vi "Receive Response.vi"(8 "error in":errorcluster, 10 "Response":string, 11 "PS in":refnum<class "Power Supply.lvclass">) -> (0 "error out":errorcluster, 3 "PS out":refnum<class "Power Supply.lvclass">)   [LabVIEW 2019, in "Power Supply.lvlib" / "Power Supply.lvclass"]
uses:
  Power Supply.lvclass
  C:/Program Files (x86)/National Instruments/LabVIEW 2019/vi.lib/ActorFramework/Actor/Actor.lvclass
  Power Supply.lvclass/Power Supply.ctl
  Serial/Serial Messages/Write Msg/Write Msg.lvclass/Write Msg.ctl
  <vilib>/ActorFramework/Message Enqueuer/Message Enqueuer.lvclass/Message Enqueuer.ctl
  <vilib>/ActorFramework/Actor/Actor.lvclass/Actor.ctl
  Power Supply Messages/PS Dataset Msg/PS Dataset Msg.lvclass/PS Dataset Msg.ctl
  <vilib>/ActorFramework/Message Enqueuer/Enqueue.vi
  Serial/Serial Messages/Write Msg/Write Msg.lvclass
  C:/Program Files (x86)/National Instruments/LabVIEW 2019/vi.lib/ActorFramework/Message/Message.lvclass
  Power Supply Messages/PS Dataset Msg/PS Dataset Msg.lvclass
  <userlib>/_MGI/Application Control/MGI Get Value/MGI Get Value (String).vi
  <vilib>/ActorFramework/Message Priority Queue/Priority Enqueue.vi
  <vilib>/ActorFramework/Actor/Actor.lvclass
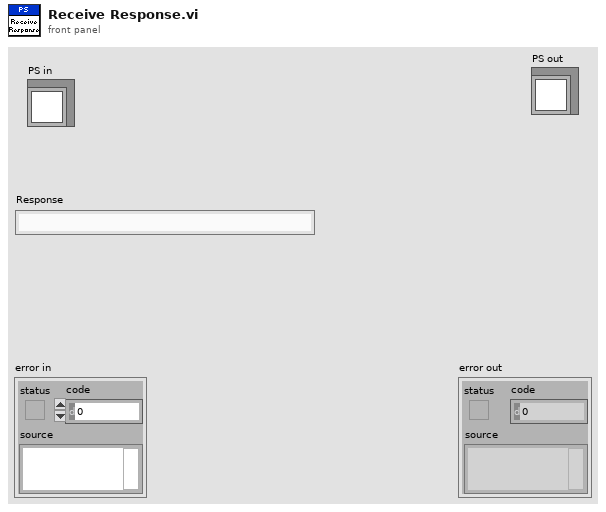
[diagram p1: front panel]
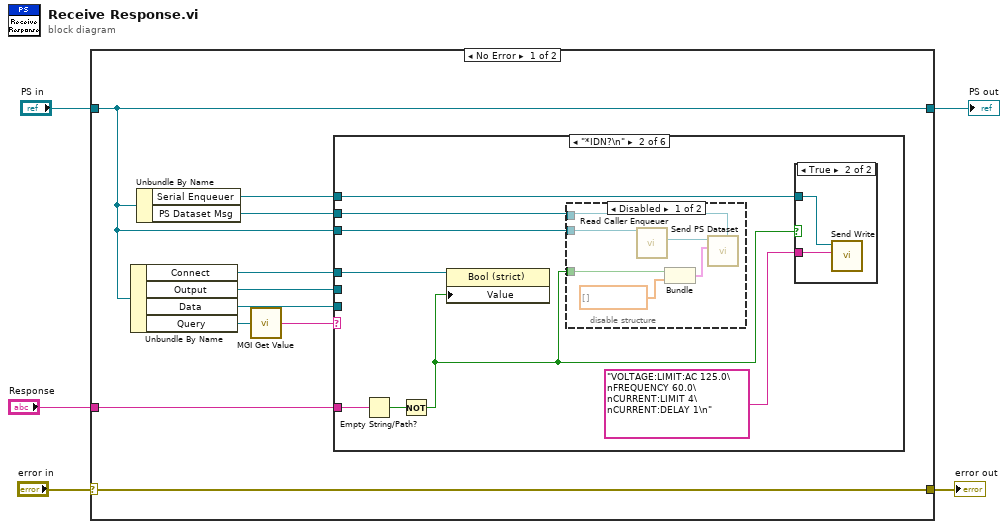
[diagram p0: block diagram]
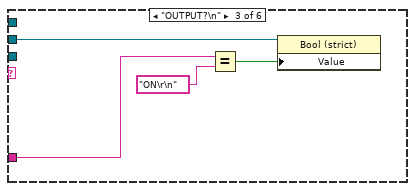
[diagram p5: hidden frame]
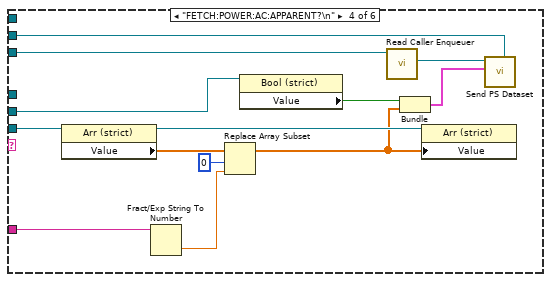
[diagram p6: hidden frame]
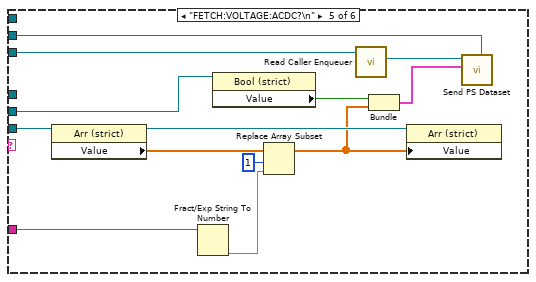
[diagram p7: hidden frame]
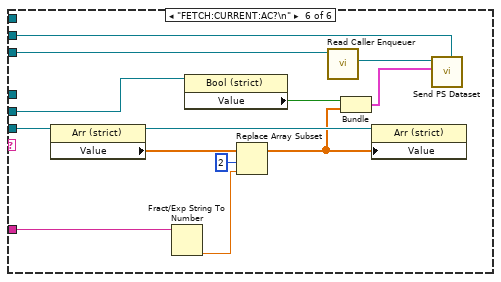
[diagram p8: hidden frame]
diagram:
  n1 = case shown="No Error" "error in" {
    selector: "error in" -> [w8 w76]
    tunnel: [w8 w76] -> w4
    tunnel: [w15 w75] -> w2
    tunnel: "PS in" -> [w15 w75]
    tunnel: "Response" -> [w14 _]
    frame No Error {
      n2 = Unbundle By Name(w15) -> ("Connect"=w12:refnum<vi>, "Output"=w11:refnum<vi>, "Data"=w13:refnum<vi>, "Query"=w7:refnum<vi>)
      n3 = Unbundle By Name(w15) -> ("Serial Enqueuer"=w10:refnum<class "Message Enqueuer.lvclass">, "PS Dataset Msg"=w9:refnum<class "PS Dataset Msg.lvclass">)
      n4 = call-poly <userlib>:"MGI Get Value.vi"("String Ref"=w7) -> ("String"=w6:string)
      n5 = case shown="\"*IDN?\\n\"" w6 {
        tunnel: w12 -> [_ w22 _ _ _ _]
        tunnel: w14 -> [_ w21 w33 w48 w61 w74]
        tunnel: w11 -> [_ _ w35 w36 w49 w62]
        tunnel: w9 -> [_ w17 _ w39 w52 w65]
        tunnel: w10 -> [_ w20 _ _ _ _]
        tunnel: w13 -> [_ _ _ w45 w58 w71]
        tunnel: w15 -> [_ w18 _ w40 w54 w67]
        frame Default {
        }
        frame "*IDN?\n" {
          n6 = Empty String/Path?(string/path=w21) -> (empty?=w23:bool)
          n7 = Not(x=w23) -> (.not. x?=w19:bool)
          n8 = property class="Bool (strict)"(reference=w22, "Value"=w19) -> ()  [unwired: 1 in, 2 out]
          n9 = disable-structure shown="Disabled" {
            disable-tunnel: w19 -> [w29 _]
            disable-tunnel: w18 -> [w28 _]
            disable-tunnel: w17 -> [w26 _]
            frame Disabled {
              n10 = call <vilib>:"Read Caller Enqueuer.vi"("Actor"=w28) -> ("Caller Enqueuer"=w25:refnum<class "Message Enqueuer.lvclass">)  [unwired: 10 in]
              n11 = Bundle(w29, dbl[] []) -> (w24:cluster{bool, dbl[]})  [unwired: 1 in]
              n12 = call "Send PS Dataset.vi"("Message Type"=w26, "PS Dataset"=w24, "Message Enqueuer"=w25) -> ()  [unwired: 7 in, 2 out]
            }
            frame Enabled {
            }
          }
          n13 = case shown="True" w19 {
            tunnel: w20 -> [_ w31]
            tunnel: "VOLTAGE:LIMIT:AC 125.0\nFREQUENCY 60.0\nCURRENT:LIMIT 4\nCURRENT:DELAY 1\n" ("Command") -> [_ w30]
            frame False {
            }
            frame True {
              n14 = call "Send Write.vi"("Command"=w30, "Message Enqueuer"=w31) -> ()  [unwired: 8 in, 2 out]
            }
          }
        }
        frame "OUTPUT?\n" {
          n15 = Equal?(x=w33, y="ON\r\n" ("Command")) -> (x = y?=w34:bool)
          n16 = property class="Bool (strict)"(reference=w35, "Value"=w34) -> ()  [unwired: 1 in, 2 out]
        }
        frame "FETCH:POWER:AC:APPARENT?\n" {
          n17 = property class="Arr (strict)"(reference=w45) -> (reference out=w44:refnum<vi>, "Value"=w43:dbl[])  [unwired: 1 in, 1 out]
          n18 = Fract/Exp String To Number(string=w48) -> (number=w46:dbl)  [unwired: 3 in, 1 out]
          n19 = Replace Array Subset(array=w43, new element=w46, index=0) -> (w41:dbl[])
          n20 = property class="Bool (strict)"(reference=w36) -> ("Value"=w42:bool)  [unwired: 1 in, 2 out]
          n21 = call <vilib>:"Read Caller Enqueuer.vi"("Actor"=w40) -> ("Caller Enqueuer"=w38:refnum<class "Message Enqueuer.lvclass">)  [unwired: 10 in]
          n22 = Bundle("Value"=w42, "Value"=w41) -> (w37:cluster{"Value":bool, "Value":dbl[]})  [unwired: 1 in]
          n23 = property class="Arr (strict)"(reference=w44, "Value"=w41) -> ()  [unwired: 1 in, 2 out]
          n24 = call "Send PS Dataset.vi"("Message Type"=w39, "PS Dataset"=w37, "Message Enqueuer"=w38) -> ()  [unwired: 7 in, 2 out]
        }
        frame "FETCH:VOLTAGE:ACDC?\n" {
          n25 = property class="Arr (strict)"(reference=w58) -> (reference out=w57:refnum<vi>, "Value"=w56:dbl[])  [unwired: 1 in, 1 out]
          n26 = Fract/Exp String To Number(string=w61) -> (number=w59:dbl)  [unwired: 3 in, 1 out]
          n27 = property class="Bool (strict)"(reference=w49) -> ("Value"=w53:bool)  [unwired: 1 in, 2 out]
          n28 = Replace Array Subset(array=w56, new element=w59, index=1) -> (w55:dbl[])
          n29 = call <vilib>:"Read Caller Enqueuer.vi"("Actor"=w54) -> ("Caller Enqueuer"=w51:refnum<class "Message Enqueuer.lvclass">)  [unwired: 10 in]
          n30 = Bundle("Value"=w53, "Value"=w55) -> (w50:cluster{"Value":bool, "Value":dbl[]})  [unwired: 1 in]
          n31 = property class="Arr (strict)"(reference=w57, "Value"=w55) -> ()  [unwired: 1 in, 2 out]
          n32 = call "Send PS Dataset.vi"("Message Type"=w52, "PS Dataset"=w50, "Message Enqueuer"=w51) -> ()  [unwired: 7 in, 2 out]
        }
        frame "FETCH:CURRENT:AC?\n" {
          n33 = property class="Arr (strict)"(reference=w71) -> (reference out=w70:refnum<vi>, "Value"=w69:dbl[])  [unwired: 1 in, 1 out]
          n34 = Fract/Exp String To Number(string=w74) -> (number=w72:dbl)  [unwired: 3 in, 1 out]
          n35 = property class="Bool (strict)"(reference=w62) -> ("Value"=w68:bool)  [unwired: 1 in, 2 out]
          n36 = Replace Array Subset(array=w69, new element=w72, index=2) -> (w66:dbl[])
          n37 = call <vilib>:"Read Caller Enqueuer.vi"("Actor"=w67) -> ("Caller Enqueuer"=w64:refnum<class "Message Enqueuer.lvclass">)  [unwired: 10 in]
          n38 = Bundle("Value"=w68, "Value"=w66) -> (w63:cluster{"Value":bool, "Value":dbl[]})  [unwired: 1 in]
          n39 = property class="Arr (strict)"(reference=w70, "Value"=w66) -> ()  [unwired: 1 in, 2 out]
          n40 = call "Send PS Dataset.vi"("Message Type"=w65, "PS Dataset"=w63, "Message Enqueuer"=w64) -> ()  [unwired: 7 in, 2 out]
        }
      }
    }
    frame Error {
    }
  }
  "error out" <- w4
  "PS out" <- w2
